vi "Is an Actor Test.vi"() -> ()   [LabVIEW 2023, in "Message Maker.lvclass"]
uses:
  Message Maker.lvclass
  Message Recipient Type.ctl
panel:
  out "Actor/Interfaces FQNs":string[](array[string])
  out "Array":T1[](array[typedef])
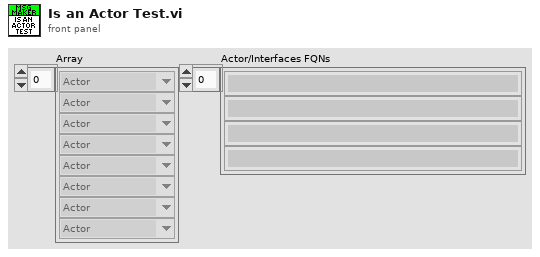
[diagram p1: front panel]
types:
  T1 = typedef "Message Maker.lvclass/Message Recipient Type.ctl" = enum16{"Actor", "Interface"}
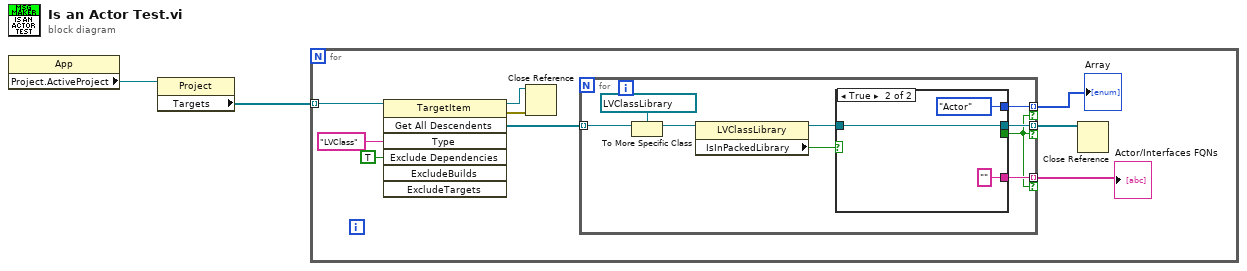
[diagram p0: block diagram]
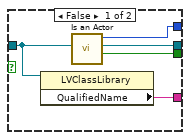
[diagram p2: hidden frame]
diagram:
  n1 = property class="App"() -> ("Project.ActiveProject"=w1:refnum<vi>)  [unwired: 2 in, 2 out]
  n2 = property class="Project"(reference=w1) -> ("Targets"=w2:refnum<vi>[])  [unwired: 1 in, 2 out]
  n3 = for {
    tunnel: w2 -> [w11] mode=indexing
    n4 = invoke class="TargetItem" method="Get All Descendents"(reference=w11, "Type"="LVClass", "Exclude Dependencies"=TRUE ("ExcludeDependencies")) -> (reference out=w7:refnum<vi>, error out=w8:errorcluster, "All Descendents"=w9:refnum<vi>[])  [unwired: 4 in, 4 out]
    n5 = Close Reference(reference=w7, error in (no error)=w8) -> ()  [unwired: 1 out]
    n6 = for {
      tunnel: w9 -> [w20] mode=indexing
      tunnel: [w17] -> w5 mode=indexing if=w12
      tunnel: [w14] -> w4 mode=indexing if=w12
      tunnel: [w13] -> w3 mode=indexing if=w12
      n7 = To More Specific Class(target class=refnum<vi> refnum ("reference out"), reference=w20) -> (specific class reference=w18:refnum<vi>)  [unwired: 1 in, 1 out]
      n8 = property class="LVClassLibrary"(reference=w18) -> (reference out=w16:refnum<vi>, "IsInPackedLibrary"=w15:bool)  [unwired: 1 in, 1 out]
      n9 = case shown="True" w15 {
        tunnel: [w25 w28] -> w17
        tunnel: [w24 _] -> w12
        tunnel: w16 -> [w22 w28]
        tunnel: [w23 Message_Recipient_Type."Actor" ("Message Recipient Type")] -> w14
        tunnel: [w21 "" ("QualifiedName")] -> w13
        frame False {
          n10 = property class="LVClassLibrary"(reference=w22) -> ("QualifiedName"=w21:string)  [unwired: 1 in, 2 out]
          n11 = call "Is an Actor.vi"("Class in"=w22) -> ("Is Actor/Interface?"=w24:bool, "Class out"=w25:refnum<vi>, "Message Recipient Type"=w23:T1)  [unwired: 7 in, 1 out]
        }
        frame True {
        }
      }
    }
    "Array" <- w4
    "Actor/Interfaces FQNs" <- w3
    n12 = Close Reference(reference=w5) -> ()  [unwired: 1 in, 1 out]
  }
